vi "ReportHead_A131258.vi"(8 "error in (no error)":errorcluster caption="错误输入（无错误）", 11 "产品状态":string) -> (0 "error out":errorcluster caption="错误输出", 3 "report out":refnum<class "NI_report.lvclass"> caption="报表输出")   [LabVIEW 2020]
uses:
  <vilib>/Utility/NIReport.llb/NI_report.lvclass
  <vilib>/addons/_office/_exclsub.llb/font.ctl
  Database/Global1.vi
  <vilib>/addons/_office/NI_ReportGenerationToolkit.lvlib
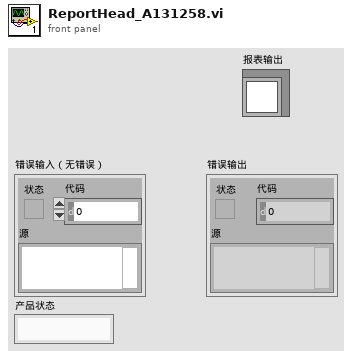
[diagram p1: front panel]
types:
  T1 = cluster{"操作者编号":string, "操作者姓名":string, "操作者权限":string, "联机状态":string, "产品型号":string, "产品状态":string}
  T2 = cluster{"top":dbl, "left":dbl, "right":dbl, "bottom":dbl}
  T3 = cluster{"Charset (-1)":i16, "Weight (-1)":i16, "Name":string, "Size":string}
  T4 = cluster{"Italic":enum16{"Italic Unchanged", "Italic On", "Italic Off"}, "Strike Through":enum16{"Strike Through Unchanged", "Strike Through On", "Strike Through Off"}, "Underline":enum16{"Underline Unchanged", "Underline On", "Underline Off"}, "Bold":enum16{"Bold Unchanged", "Bold On", "Bold Off"}}
  T5 = typedef "NI_ReportGenerationToolkit.lvlib/font.ctl" = cluster{"font name":string, "font size":dbl, "bold":u16, "italic":u16, "underline":u16, "strike through":u16, "font color":u32}
  T6 = enum16{"maximized", "minimized", "normal", "no change"}
  T7 = enum16{"Standard Report", "HTML", "Word", "Excel"}
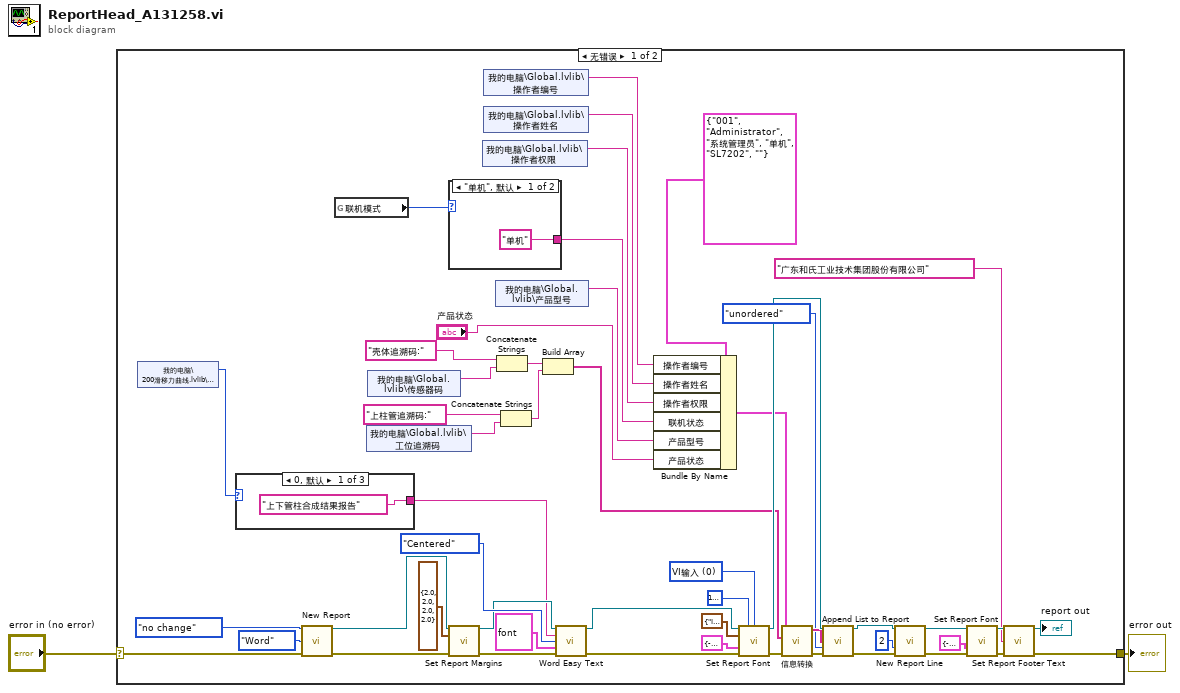
[diagram p0: block diagram]
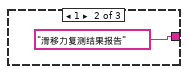
[diagram p2: hidden frame]
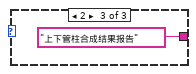
[diagram p3: hidden frame]
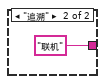
[diagram p4: hidden frame]
diagram:
  n1 = case shown="无错误" "error in (no error)" {
    selector: "error in (no error)" -> [w26 w58]
    tunnel: [w22 w58] -> w1
    frame No Error {
      w45 = u16 0 items=["VI输入", "字体对话框"] ("font settings source")
      n2 = shared-variable "我的电脑\\200滑移力曲线.lvlib\\备用_5"() -> (w3:u16)  [unwired: 1 in, 1 out]
      n3 = case shown="0, 默认" w3 {
        tunnel: ["上下管柱合成结果报告" ("text") "滑移力复测结果报告" ("text") "上下管柱合成结果报告" ("text")] -> w8
        frame 0, Default {
        }
        frame 1 {
        }
        frame 2 {
        }
      }
      n4 = call <vilib>:"New Report.vi"("window state (normal)"=T6."no change", "report type"=T7."Word", "error in (no error)"=w26) -> ("report out"=w39:refnum<class "NI_report.lvclass">, "error out"=w36:errorcluster)  [unwired: 11 in]
      n5 = global read "Global1.vi" "联机模式"() -> (w4:enum16{"单机", "追溯"})
      n6 = shared-variable "我的电脑\\Global.lvlib\\工位追溯码"() -> (w7:string)  [unwired: 1 in, 1 out]
      n7 = shared-variable "我的电脑\\Global.lvlib\\传感器码"() -> (w12:string)  [unwired: 1 in, 1 out]
      n8 = case shown="\"单机\", 默认" w4 {
        tunnel: ["单机" "联机"] -> w16
        frame "单机", Default {
        }
        frame "追溯" {
        }
      }
      n9 = call-dynamic "Set Report Margins.vi"("report in"=w39, "margins (1.00)"=T2 {"top"=2.0, "left"=2.0, "right"=2.0, "bottom"=2.0}, "error in (no error)"=w36) -> ("report out"=w38:refnum<class "NI_report.lvclass">, "error out"=w37:errorcluster)  [unwired: 10 in, 1 out]
      n10 = shared-variable "我的电脑\\Global.lvlib\\操作者权限"() -> (w19:string)  [unwired: 1 in, 1 out]
      n11 = shared-variable "我的电脑\\Global.lvlib\\操作者编号"() -> (w20:string)  [unwired: 1 in, 1 out]
      n12 = shared-variable "我的电脑\\Global.lvlib\\操作者姓名"() -> (w18:string)  [unwired: 1 in, 1 out]
      n13 = shared-variable "我的电脑\\Global.lvlib\\产品型号"() -> (w17:string)  [unwired: 1 in, 1 out]
      n14 = Concatenate Strings("壳体追溯码:", w12) -> (w11:string)
      n15 = Concatenate Strings("上柱管追溯码:", w7) -> (w5:string)
      n16 = Build Array(w11, w5) -> (w10:string[])
      n17 = call <vilib>:"Word Easy Text.vi"("report in"=w38, "text"=w8, "alignment (left)"=enum16{"Left", "Centered", "Right", "Justify"}."Centered", "font"=T5 {"font name"="楷体", "font size"=26.0, "bold"=1, "italic"=2, "underline"=2, "strike through"=2, "font color"=16777228}, "error in (no error)"=w37) -> ("report out"=w47:refnum<class "NI_report.lvclass">, "error out"=w46:errorcluster)  [unwired: 8 in, 1 out]
      n18 = Bundle By Name(cluster=T1 {"操作者编号"="001", "操作者姓名"="Administrator", "操作者权限"="系统管理员", "联机状态"="单机", "产品型号"="SL7202", "产品状态"=""} ("测试信息"), "操作者编号"=w20, "操作者姓名"=w18, "操作者权限"=w19, "联机状态"=w16, "产品型号"=w17, "产品状态"="产品状态") -> (w14:T1)
      n19 = call-dynamic "Set Report Font.vi"("report in"=w47, "text color (unchanged)"=u32 16777224, "font settings source (VI Inputs)"=w45, "text options"=T4 {"Italic"=enum."Italic Off", "Strike Through"=enum."Strike Through Unchanged", "Underline"=enum."Underline Off", "Bold"=enum."Bold Off"}, "font settings"=T3 {"Charset (-1)"=-1, "Weight (-1)"=-1, "Name"="微软雅黑 Light", "Size"="12 "}, "error in (no error)"=w46) -> ("report out"=w34:refnum<class "NI_report.lvclass">, "error out"=w25:errorcluster)  [unwired: 7 in, 1 out]
      n20 = call "信息转换.vi"("错误输入（无错误）"=w25, "追溯码"=w10, "测试信息"=w14) -> ("错误输出"=w24:errorcluster, "信息输出"=w27:string[])  [unwired: 7 in]
      n21 = call-dynamic "Append List to Report.vi"("report in"=w34, "list elements"=w27, "list type (ordered)"=enum16{"unordered", "ordered"}."unordered", "error in (no error)"=w24) -> ("report out"=w29:refnum<class "NI_report.lvclass">, "error out"=w28:errorcluster)  [unwired: 8 in, 2 out]
      n22 = call-dynamic "New Report Line.vi"("report in"=w29, "number of lines (1)"=2, "error in (no error)"=w28) -> ("report out"=w32:refnum<class "NI_report.lvclass">, "error out"=w33:errorcluster)  [unwired: 11 in]
      n23 = call-dynamic "Set Report Font.vi"("report in"=w32, "font settings"=T3 {"Charset (-1)"=-1, "Weight (-1)"=-1, "Name"="楷体", "Size"="9 "}, "error in (no error)"=w33) -> ("report out"=w43:refnum<class "NI_report.lvclass">, "error out"=w42:errorcluster)  [unwired: 10 in, 1 out]
      n24 = call-dynamic "Set Report Footer Text.vi"("report in"=w43, "center footer text"="广东和氏工业技术集团股份有限公司", "error in (no error)"=w42) -> ("report out"=→"report out":refnum<class "NI_report.lvclass">, "error out"=w22:errorcluster)  [unwired: 11 in]
    }
    frame Error {
    }
  }
  "error out" <- w1
